vi "Create Default Measurement Database.vi"(8 "error in (no error)":errorcluster, 11 "QPA Measurement in":refnum<class "QPA Measurement.lvclass">) -> (0 "error out":errorcluster, 3 "QPA Measurement out":refnum<class "QPA Measurement.lvclass">)   [LabVIEW 2016, in "QPA Measurement.lvlib" / "QPA Measurement.lvclass"]
uses:
  QPA Measurement.lvclass
  C:/Projects/STS/Common/Sequence Automation/Plugins/Measurement Interface.lvlibp/Measurement Interface.lvclass
  QPA Measurement.lvclass/QPA Measurement.ctl
  Plugins/Measurement Interface.lvlibp/Private Methods/Active Sequence File/Read Active Sequence File.vi
  Plugins/TestStand API Tools (TSAT).lvlibp/Sequence File Actions/TSAT Sequence File Actions.lvlib
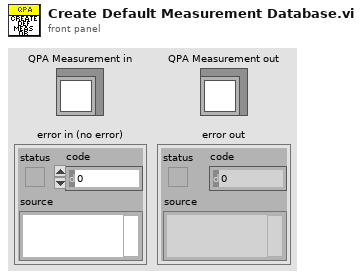
[diagram p1: front panel]
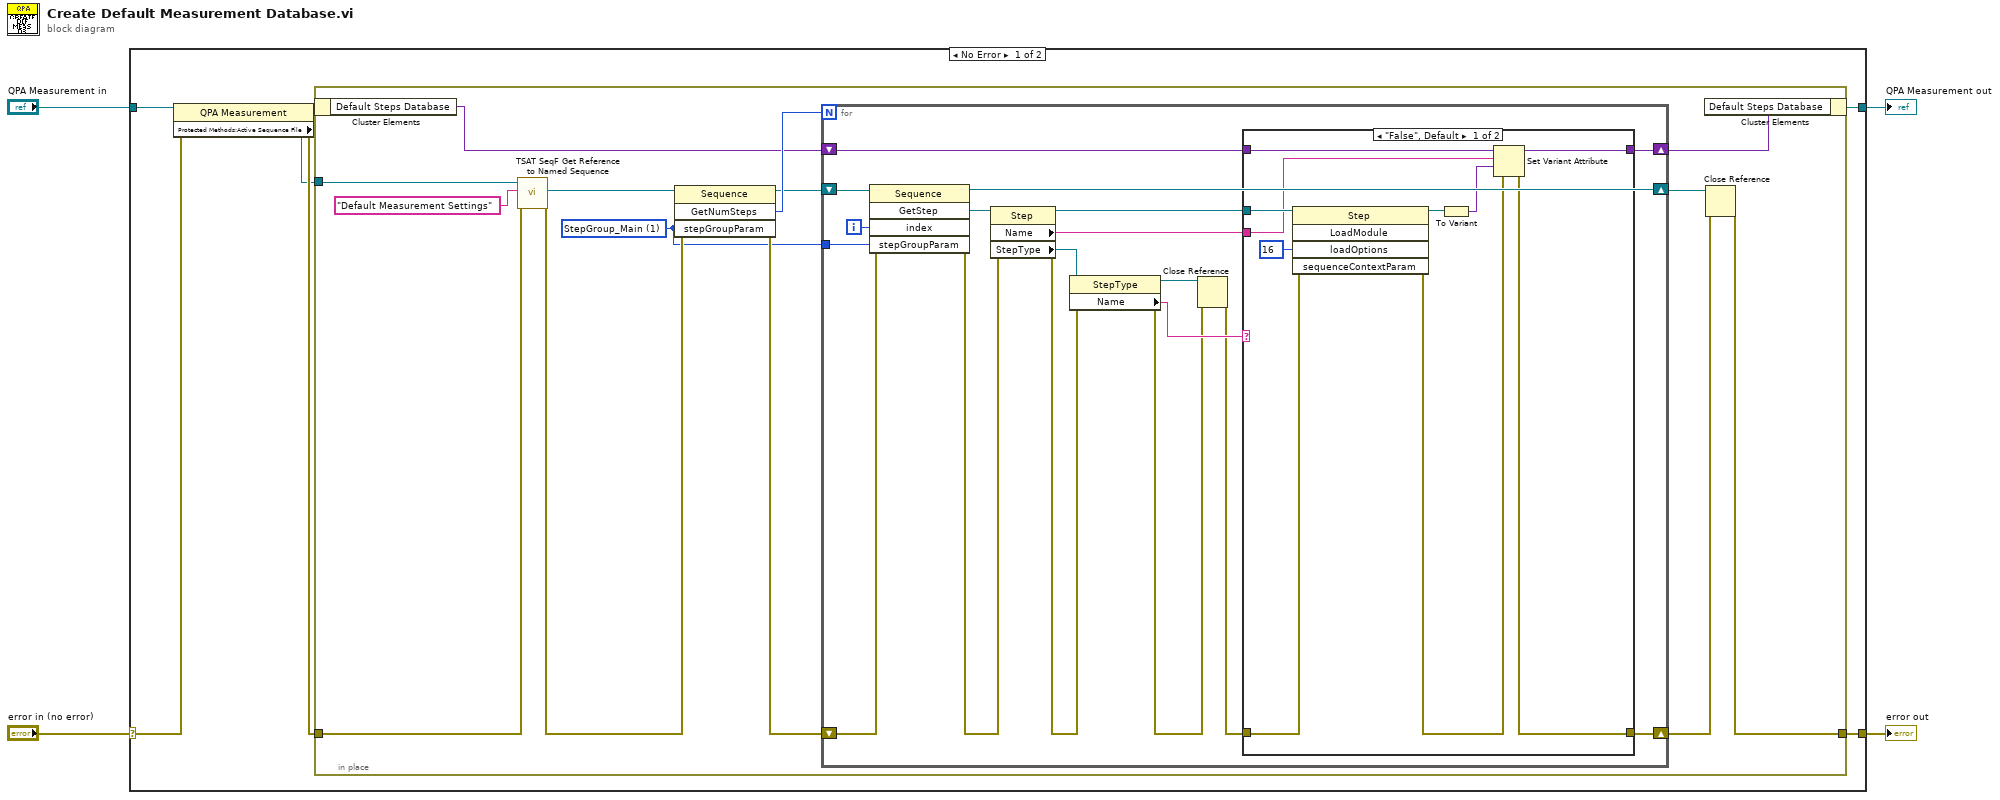
[diagram p0: block diagram]
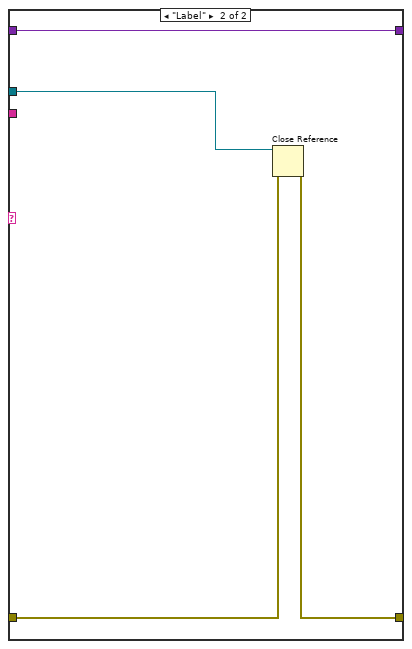
[diagram p2: hidden frame]
diagram:
  n1 = case shown="No Error" "error in (no error)" {
    selector: "error in (no error)" -> [w11 w59]
    tunnel: [w5 w59] -> w3
    tunnel: [w6 w58] -> w1
    tunnel: "QPA Measurement in" -> [w9 w58]
    frame No Error {
      n2 = property class="QPA Measurement"(reference=w9, error in=w11) -> (reference out=w8:refnum<class "QPA Measurement.lvclass">, error out=w10:errorcluster, "Protected Methods:Active Sequence File"=w7:refnum<k7>)
      n3 = in-place {
        in-place-border: w10 -> [w24]
        in-place-border: w7 -> [w25]
        in-place-border: [w12] -> w5
        w17 = 1 items=["StepGroup_Setup", "StepGroup_Main", "StepGroup_Cleanup"] ("stepGroupParam")
        n4 = in-place-cluster #1(w8) -> ("Default Steps Database"=w16:variant)
        n5 = call "TSAT SeqF Get Reference to Named Sequence.vi"("Error In"=w24, "Seqeunce to Retrieve"="Default Measurement Settings", "Sequence File In"=w25) -> ("Error Out"=w21:errorcluster, "Named Sequence"=w22:refnum<k7>)  [unwired: 6 in, 1 out]
        n6 = invoke class="Sequence" method="GetNumSteps"(reference=w22, error in=w21, "stepGroupParam"=w17) -> (reference out=w19:refnum<k7>, error out=w18:errorcluster, "GetNumSteps"=w20:i32)  [unwired: 1 in, 1 out]
        n7 = for {
          N: w20 -> [_]
          shift-right: [w37] -> w14
          shift-left: w19 -> [w43]
          shift-right: [w31] -> w13
          shift-left: w18 -> [w41]
          tunnel: w17 -> [w40]
          shift-right: [w26] -> w15
          shift-left: w16 -> [w27]
          i -> [w42]
          n8 = invoke class="Sequence" method="GetStep"(reference=w43, error in=w41, "index"=w42, "stepGroupParam"=w40) -> (reference out=w37:refnum<k7>, error out=w38:errorcluster, "GetStep"=w39:refnum<k7>)  [unwired: 1 in, 2 out]
          n9 = property class="Step"(reference=w39, error in=w38) -> (reference out=w32:refnum<k7>, error out=w36:errorcluster, "Name"=w28:string, "StepType"=w29:refnum<k7>)
          n10 = property class="StepType"(reference=w29, error in=w36) -> (reference out=w34:refnum<k7>, error out=w33:errorcluster, "Name"=w35:string)
          n11 = Close Reference(reference=w34, error in (no error)=w33) -> (error out=w30:errorcluster)
          n12 = case shown="\"False\", Default" w35 {
            tunnel: w32 -> [w52 w57]
            tunnel: [w49 w55] -> w31
            tunnel: w30 -> [w46 w56]
            tunnel: w28 -> [w50 _]
            tunnel: w27 -> [w53 w54]
            tunnel: [w48 w54] -> w26
            frame "False", Default {
              n13 = invoke class="Step" method="LoadModule"(reference=w52, error in=w46, "loadOptions"=16) -> (reference out=w47:refnum<k7>, error out=w45:errorcluster)  [unwired: 2 in, 3 out]
              n14 = To Variant(anything=w47) -> (Variant=w51:variant)
              n15 = Set Variant Attribute(Variant=w53, name=w50, value=w51, error in=w45) -> (Variant out=w48:variant, error out=w49:errorcluster)  [unwired: 1 out]
            }
            frame "Label" {
              n16 = Close Reference(reference=w57, error in (no error)=w56) -> (error out=w55:errorcluster)
            }
          }
        }
        n17 = in-place-cluster #1("Default Steps Database"=w15) -> (w6:refnum<class "QPA Measurement.lvclass">)
        n18 = Close Reference(reference=w14, error in (no error)=w13) -> (error out=w12:errorcluster)
      }
    }
    frame Error {
    }
  }
  "error out" <- w3
  "QPA Measurement out" <- w1
